vi "Synchronize Caller Events.vi"(8 "error in (no error)":errorcluster, 11 "Singleton Module Admin in":refnum<class "Delacor_lib_QMH_Module Admin.lvclass">) -> (0 "error out":errorcluster, 3 "Singleton Module Admin out":refnum<class "Delacor_lib_QMH_Module Admin.lvclass">)   [LabVIEW 2017, in "CML UI.lvlib"]
doc: "Synchronize with the caller of the module through the sequence of waiting on multiple rendezvous.\n_____\nBased on Delacor QMH Project Template 4.0.0.47.\n_____\nBased on Delacor QMH Project Template 4.1.0.56."
uses:
  CML UI.lvlib
  <vilib>/Delacor/Delacor QMH/Libraries/Module Admin_class/Delacor_lib_QMH_Module Admin.lvclass
  <vilib>/Delacor/Delacor QMH/Libraries/Module Admin_class/Delacor_lib_QMH_Module Admin.lvclass/Delacor_lib_QMH_Module Admin.ctl
  <vilib>/Delacor/Delacor QMH/Libraries/Module Admin_class/Delacor_lib_QMH_Get External Launch.vi
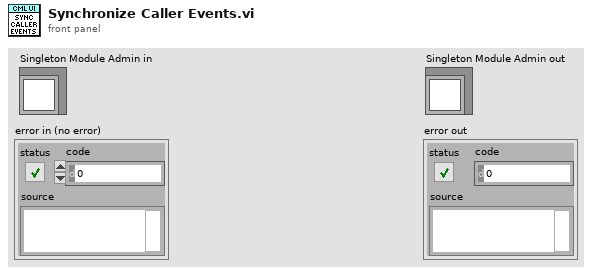
[diagram p1: front panel]
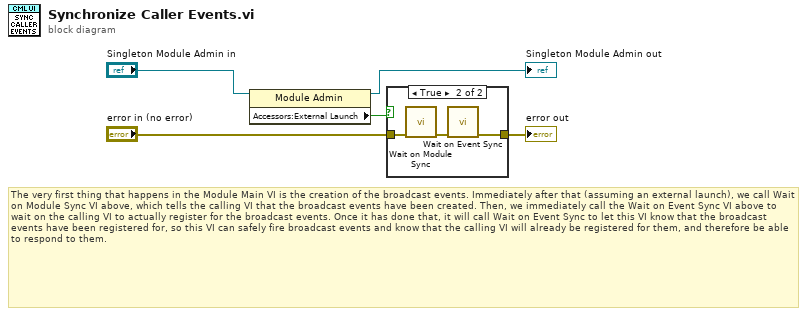
[diagram p0: block diagram]
diagram:
  # "The very first thing that happens in the Module Main VI is the creation of the broadcast events. Immediately after that (assuming an external launch), we call Wait on Module Sync VI above, which tells the calling VI that the broadcast events have been created. Then, we immediately call the Wait on Event Sync VI above to wait on the calling VI to actually register for the broadcast events. Once it has done that, it will call Wait on Event Sync to let this VI know that the broadcast events have been registered for, so this VI can safely fire broadcast events and know that the calling VI will already be registered for them, and therefore be able to respond to them."
  n1 = property on="Property Node" class="Module Admin"(reference="Singleton Module Admin in") -> (reference out=→"Singleton Module Admin out":refnum<class "Delacor_lib_QMH_Module Admin.lvclass">, "Accessors:External Launch"=w3:bool)  [unwired: 1 in, 1 out]
  n2 = case shown="True" w3 {
    tunnel: "error in (no error)" -> [w6 w9]
    tunnel: [w6 w7] -> w5
    frame False {
    }
    frame True {
      n3 = call "Wait on Module Sync.vi"("error in (no error)"=w9) -> ("error out"=w8:errorcluster)  [unwired: 10 in]
      n4 = call "Wait on Event Sync.vi"("error in (no error)"=w8) -> ("error out"=w7:errorcluster)  [unwired: 10 in]
    }
  }
  "error out" <- w5
